vi "Lab Panel V4.86.vi"() -> ()   [LabVIEW 2013] (continued)
                        n565 = Create Folder(path (use dialog)=w897) -> (error out=w896:errorcluster)  [unwired: 2 in, 2 out]
                        n566 = global write "Global 1.vi" "LAB02-1 FILE"(w883) -> ()
                        n567 = call <vilib>:"Clear Errors.vi"("error in (no error)"=w896) -> ()  [unwired: 6 in, 1 out]
                      }
                      frame #1 {
                        (unwired) FALSE
                        n568 = String To Path(string=w907) -> (path=w903:path)
                        n569 = TDMS Open(6:FALSE, 10:T18."create or replace" ("operation (0:open)"), 11:w903) -> (0:w902:errorcluster, 3:→"TDMS LAB02-1":refnum<k34>)  [unwired: 4 in]
                      }
                      frame #2 {
                        n570 = local read "SET LAB02-1"() -> (w913:T5)
                        n571 = local read "TDMS LAB02-1"() -> (w924:refnum<k34>)
                        n572 = Build Array("Testers Name", "Description", "Set Test Cycles", "T-Rise minutes", "T-Rise Deg C") -> (w914:string[])
                        n573 = Unbundle(w913) -> ("NAME"=w912:string, "DESCRIPTION"=w911:string, "CYCLES"=w910:dbl, "T-RISE mins"=w909:dbl, "T-RISE deg C"=w908:dbl)
                        n574 = Number To Decimal String(number=w910) -> (decimal integer string=w923:string)  [unwired: 1 in]
                        n575 = Number To Decimal String(number=w909) -> (decimal integer string=w922:string)  [unwired: 1 in]
                        n576 = Number To Decimal String(number=w908) -> (decimal integer string=w921:string)  [unwired: 1 in]
                        n577 = Build Array(w912, w911, w923, w922, w921) -> (w920:string[])
                        n578 = TDMS Set Properties(5:w920, 7:w914, 11:w924) -> ()  [unwired: 3 in, 4 out]
                      }
                      frame #3 {
                        n579 = local read "DISP LAB02-1"() -> (w929:T4)
                        n580 = Concatenate Strings("LAB02-1  ", w928) -> (w930:string)
                        n581 = Two Button Dialog(message=w930, 1:w926, 2:w927) -> (T button?=w932:bool)
                        n582 = case shown="True" w932 {
                          tunnel: w929 -> [w939 w940]
                          tunnel: [w939 w940] -> w936
                          tunnel: [w938 w941] -> w935
                          tunnel: [w937 w941] -> w934
                          frame False {
                            n583 = Unbundle(w939) -> ("CYCLE"=w938:dbl, "MINS"=w937:dbl)  [unwired: 1 out]
                          }
                          frame True {
                            w941 = 0.0
                          }
                        }
                        n584 = Bundle(cluster=w936, "CYCLE"=w935, "MINS"=w934, "STATUS"="RUN") -> (w925:T4)
                        n585 = local write "DISP LAB02-1"(w925) -> ()
                      }
                      frame #4 {
                        n586 = local read "SIG LAB02-1"() -> (w944:T2)
                        n587 = local read "TEMP START LAB02-1"() -> (w946:cluster{"TL":dbl, "TN":dbl})
                        n588 = Unbundle(w944) -> ("Tmp Live"=w943:dbl, "Tmp Neut"=w942:dbl)  [unwired: 3 out]
                        n589 = Bundle(cluster=w946, "TL"=w943, "TN"=w942) -> (w945:cluster{"TL":dbl, "TN":dbl})
                        n590 = local write "TEMP START LAB02-1"(w945) -> ()
                      }
                    }
                  }
                }
              }
              event "RUN LAB02-2": Value Change {
                n591 = event-data() -> ("NewVal"=w950:bool)  [unwired: 1 in, 5 out]
                n592 = local write "run lab02-2"(w950) -> ()
                n593 = case shown="True" w950 {
                  tunnel: w956 -> [_ w992]
                  tunnel: w955 -> [_ w991]
                  tunnel: w953 -> [w958 w990]
                  tunnel: w954 -> [_ w989]
                  tunnel: w952 -> [_ w988]
                  tunnel: [w957 w987] -> w951
                  tunnel: w949 -> [_ w986]
                  tunnel: w948 -> [_ w985]
                  tunnel: w947 -> [_ w984]
                  frame False {
                    # "stop test"
                    n594 = stacked-sequence {
                      tunnel: w958 -> [w967 _]
                      tunnel: [w959 _] -> w957
                      frame #0 {
                        n595 = local read "DISP LAB02-2"() -> (w966:T4)
                        n596 = Unbundle(w966) -> ("CYCLE"=w964:dbl, "MINS"=w965:dbl)  [unwired: 1 out]
                        n597 = case shown="\"CYCLE TEST\"" w967 {
                          tunnel: w965 -> [_ _ w974]
                          tunnel: w964 -> [w972 w973 _]
                          tunnel: [w972 w973 w974] -> w963
                          frame "CHART TEST", Default {
                          }
                          frame "CYCLE TEST" {
                          }
                          frame "T-RISE TEST" {
                          }
                        }
                        n598 = local read "TDMS LAB02-2"() -> (w971:refnum<k34>)
                        n599 = Build Array("STOPPED") -> (w968:string[])
                        n600 = Build Array(w963) -> (w962:dbl[])
                        n601 = TDMS Write(0:w971, 5:"TEST RESULT", 7:w968, 9:w962) -> (4:w960:refnum<k34>, 15:w961:errorcluster)  [unwired: 2 in, 2 out]
                        n602 = TDMS Close(8:w961, 11:w960) -> (0:w959:errorcluster)  [unwired: 1 out]
                      }
                      frame #1 {
                        n603 = local read "DISP LAB02-2"() -> (w978:T4)
                        n604 = stacked-sequence {
                          tunnel: "LAB02-2" -> [w980 w982]
                          frame #0 {
                            n605 = call "sub vi - defrag tdms v1.vi"("panel id"=w980) -> ("error out"=w979:errorcluster)  [unwired: 10 in]
                            n606 = local write "data file error"(w979) -> ()
                          }
                          frame #1 {
                            n607 = call "Save data file to network drive v2.vi"("panel id"=w982) -> ("network file save error"=w981:errorcluster)  [unwired: 9 in, 1 out]
                            n608 = local write "RESULT LAB02-2"(FALSE) -> ()
                            n609 = local write "data file error"(w981) -> ()
                          }
                        }
                        n610 = Bundle(cluster=w978, "STATUS"="STOP") -> (w976:T4)  [unwired: 2 in]
                        n611 = local write "DISP LAB02-2"(w976) -> ()
                      }
                    }
                  }
                  frame True {
                    # "start new test and create test file"
                    n612 = stacked-sequence {
                      seq-local: [w993 _ _ _ _] -> [_ w1017 _ _ _]
                      tunnel: w992 -> [w998 _ _ _ _]
                      tunnel: w991 -> [w995 _ _ _ _]
                      tunnel: w990 -> [w1008 _ _ _ _]
                      tunnel: w989 -> [w1001 _ _ _ _]
                      tunnel: w988 -> [w996 _ _ _ _]
                      tunnel: [_ w1012 _ _ _] -> w987
                      tunnel: w986 -> [_ _ _ w1038 _]
                      tunnel: w985 -> [_ _ _ w1037 _]
                      tunnel: w984 -> [_ _ _ w1036 _]
                      frame #0 {
                        w994 = "\\"
                        n613 = local read "SET LAB02-2"() -> (w1003:T5)
                        n614 = case shown="\"CYCLE TEST\"" w1008 {
                          tunnel: ["L02-2-CHART TEST-" "L02-2-CYCLE TEST-" "L02-2-T-RISE TEST-"] -> w1004
                          frame "CHART TEST", Default {
                          }
                          frame "CYCLE TEST" {
                          }
                          frame "T-RISE TEST" {
                          }
                        }
                        n615 = Unbundle(w1003) -> ("DESCRIPTION"=w1002:string)  [unwired: 4 out]
                        n616 = Concatenate Strings(w998, "\\", w996, w994, w995, w994) -> (w1005:string)
                        n617 = String To Path(string=w1005) -> (path=w1007:path)
                        n618 = Concatenate Strings(w1005, w1004, w1002, "-", w1001, ".tdms") -> (w993:string)
                        n619 = Create Folder(path (use dialog)=w1007) -> (error out=w1006:errorcluster)  [unwired: 2 in, 2 out]
                        n620 = global write "Global 1.vi" "LAB02-2 FILE"(w993) -> ()
                        n621 = call <vilib>:"Clear Errors.vi"("error in (no error)"=w1006) -> ()  [unwired: 6 in, 1 out]
                      }
                      frame #1 {
                        (unwired) FALSE
                        n622 = String To Path(string=w1017) -> (path=w1013:path)
                        n623 = TDMS Open(6:FALSE, 10:T18."create or replace" ("operation (0:open)"), 11:w1013) -> (0:w1012:errorcluster, 3:→"TDMS LAB02-2":refnum<k34>)  [unwired: 4 in]
                      }
                      frame #2 {
                        n624 = local read "SET LAB02-2"() -> (w1023:T5)
                        n625 = local read "TDMS LAB02-2"() -> (w1034:refnum<k34>)
                        n626 = Build Array("Testers Name", "Description", "Set Test Cycles", "T-Rise minutes", "T-Rise Deg C") -> (w1024:string[])
                        n627 = Unbundle(w1023) -> ("NAME"=w1022:string, "DESCRIPTION"=w1021:string, "CYCLES"=w1020:dbl, "T-RISE mins"=w1019:dbl, "T-RISE deg C"=w1018:dbl)
                        n628 = Number To Decimal String(number=w1020) -> (decimal integer string=w1033:string)  [unwired: 1 in]
                        n629 = Number To Decimal String(number=w1019) -> (decimal integer string=w1032:string)  [unwired: 1 in]
                        n630 = Number To Decimal String(number=w1018) -> (decimal integer string=w1031:string)  [unwired: 1 in]
                        n631 = Build Array(w1022, w1021, w1033, w1032, w1031) -> (w1030:string[])
                        n632 = TDMS Set Properties(5:w1030, 7:w1024, 11:w1034) -> ()  [unwired: 3 in, 4 out]
                      }
                      frame #3 {
                        n633 = local read "DISP LAB02-2"() -> (w1039:T4)
                        n634 = Concatenate Strings("LAB02-2  ", w1038) -> (w1040:string)
                        n635 = Two Button Dialog(message=w1040, 1:w1036, 2:w1037) -> (T button?=w1042:bool)
                        n636 = case shown="True" w1042 {
                          tunnel: w1039 -> [w1049 w1050]
                          tunnel: [w1049 w1050] -> w1046
                          tunnel: [w1048 w1051] -> w1045
                          tunnel: [w1047 w1051] -> w1044
                          frame False {
                            n637 = Unbundle(w1049) -> ("CYCLE"=w1048:dbl, "MINS"=w1047:dbl)  [unwired: 1 out]
                          }
                          frame True {
                            w1051 = 0.0
                          }
                        }
                        n638 = Bundle(cluster=w1046, "CYCLE"=w1045, "MINS"=w1044, "STATUS"="RUN") -> (w1035:T4)
                        n639 = local write "DISP LAB02-2"(w1035) -> ()
                      }
                      frame #4 {
                        n640 = local read "SIG LAB02-2"() -> (w1054:T2)
                        n641 = local read "TEMP START LAB02-2"() -> (w1056:cluster{"TL":dbl, "TN":dbl})
                        n642 = Unbundle(w1054) -> ("Tmp Live"=w1053:dbl, "Tmp Neut"=w1052:dbl)  [unwired: 3 out]
                        n643 = Bundle(cluster=w1056, "TL"=w1053, "TN"=w1052) -> (w1055:cluster{"TL":dbl, "TN":dbl})
                        n644 = local write "TEMP START LAB02-2"(w1055) -> ()
                      }
                    }
                  }
                }
              }
              event "RUN LAB03-1": Value Change {
                n645 = event-data() -> ("NewVal"=w1060:bool)  [unwired: 1 in, 5 out]
                n646 = local write "run lab03-1"(w1060) -> ()
                n647 = case shown="True" w1060 {
                  tunnel: w1066 -> [_ w1102]
                  tunnel: w1065 -> [_ w1101]
                  tunnel: w1063 -> [w1068 w1100]
                  tunnel: w1064 -> [_ w1099]
                  tunnel: w1062 -> [_ w1098]
                  tunnel: [w1067 w1097] -> w1061
                  tunnel: w1059 -> [_ w1096]
                  tunnel: w1058 -> [_ w1095]
                  tunnel: w1057 -> [_ w1094]
                  frame False {
                    # "stop test"
                    n648 = stacked-sequence {
                      tunnel: w1068 -> [w1077 _]
                      tunnel: [w1069 _] -> w1067
                      frame #0 {
                        n649 = local read "DISP LAB03-1"() -> (w1076:T4)
                        n650 = Unbundle(w1076) -> ("CYCLE"=w1074:dbl, "MINS"=w1075:dbl)  [unwired: 1 out]
                        n651 = case shown="\"CYCLE TEST\"" w1077 {
                          tunnel: w1075 -> [_ _ w1084]
                          tunnel: w1074 -> [w1082 w1083 _]
                          tunnel: [w1082 w1083 w1084] -> w1073
                          frame "CHART TEST", Default {
                          }
                          frame "CYCLE TEST" {
                          }
                          frame "T-RISE TEST" {
                          }
                        }
                        n652 = local read "TDMS LAB03-1"() -> (w1081:refnum<k34>)
                        n653 = Build Array("STOPPED") -> (w1078:string[])
                        n654 = Build Array(w1073) -> (w1072:dbl[])
                        n655 = TDMS Write(0:w1081, 5:"TEST RESULT", 7:w1078, 9:w1072) -> (4:w1070:refnum<k34>, 15:w1071:errorcluster)  [unwired: 2 in, 2 out]
                        n656 = TDMS Close(8:w1071, 11:w1070) -> (0:w1069:errorcluster)  [unwired: 1 out]
                      }
                      frame #1 {
                        n657 = local read "DISP LAB03-1"() -> (w1088:T4)
                        n658 = stacked-sequence {
                          tunnel: "LAB03-1" -> [w1090 w1092]
                          frame #0 {
                            n659 = call "sub vi - defrag tdms v1.vi"("panel id"=w1090) -> ("error out"=w1089:errorcluster)  [unwired: 10 in]
                            n660 = local write "data file error"(w1089) -> ()
                          }
                          frame #1 {
                            n661 = call "Save data file to network drive v2.vi"("panel id"=w1092) -> ("network file save error"=w1091:errorcluster)  [unwired: 9 in, 1 out]
                            n662 = local write "RESULT LAB03-1"(FALSE) -> ()
                            n663 = local write "data file error"(w1091) -> ()
                          }
                        }
                        n664 = Bundle(cluster=w1088, "STATUS"="STOP") -> (w1086:T4)  [unwired: 2 in]
                        n665 = local write "DISP LAB03-1"(w1086) -> ()
                      }
                    }
                  }
                  frame True {
                    # "start new test and create test file"
                    n666 = stacked-sequence {
                      seq-local: [w1103 _ _ _ _] -> [_ w1127 _ _ _]
                      tunnel: w1102 -> [w1108 _ _ _ _]
                      tunnel: w1101 -> [w1105 _ _ _ _]
                      tunnel: w1100 -> [w1118 _ _ _ _]
                      tunnel: w1099 -> [w1111 _ _ _ _]
                      tunnel: w1098 -> [w1106 _ _ _ _]
                      tunnel: [_ w1122 _ _ _] -> w1097
                      tunnel: w1096 -> [_ _ _ w1147 _]
                      tunnel: w1095 -> [_ _ _ w1146 _]
                      tunnel: w1094 -> [_ _ _ w1145 _]
                      frame #0 {
                        w1104 = "\\"
                        n667 = local read "SET LAB03-1"() -> (w1113:T5)
                        n668 = case shown="\"T-RISE TEST\"" w1118 {
                          tunnel: ["L03-1-CHART TEST-" "L03-1-CYCLE TEST-" "L03-1-T-RISE TEST-"] -> w1114
                          frame "CHART TEST", Default {
                          }
                          frame "CYCLE TEST" {
                          }
                          frame "T-RISE TEST" {
                          }
                        }
                        n669 = Unbundle(w1113) -> ("DESCRIPTION"=w1112:string)  [unwired: 4 out]
                        n670 = Concatenate Strings(w1108, "\\", w1106, w1104, w1105, w1104) -> (w1115:string)
                        n671 = String To Path(string=w1115) -> (path=w1117:path)
                        n672 = Concatenate Strings(w1115, w1114, w1112, "-", w1111, ".tdms") -> (w1103:string)
                        n673 = Create Folder(path (use dialog)=w1117) -> (error out=w1116:errorcluster)  [unwired: 2 in, 2 out]
                        n674 = global write "Global 1.vi" "LAB03-1 FILE"(w1103) -> ()
                        n675 = call <vilib>:"Clear Errors.vi"("error in (no error)"=w1116) -> ()  [unwired: 6 in, 1 out]
                      }
                      frame #1 {
                        (unwired) FALSE
                        n676 = String To Path(string=w1127) -> (path=w1123:path)
                        n677 = TDMS Open(6:FALSE, 10:T18."create or replace" ("operation (0:open)"), 11:w1123) -> (0:w1122:errorcluster, 3:→"TDMS LAB03-1":refnum<k34>)  [unwired: 4 in]
                      }
                      frame #2 {
                        n678 = local read "SET LAB03-1"() -> (w1133:T5)
                        n679 = local read "TDMS LAB03-1"() -> (w1144:refnum<k34>)
                        n680 = Build Array("Testers Name", "Description", "Set Test Cycles", "T-Rise minutes", "T-Rise Deg C") -> (w1134:string[])
                        n681 = Unbundle(w1133) -> ("NAME"=w1132:string, "DESCRIPTION"=w1131:string, "CYCLES"=w1130:dbl, "T-RISE mins"=w1129:dbl, "T-RISE deg C"=w1128:dbl)
                        n682 = Number To Decimal String(number=w1130) -> (decimal integer string=w1143:string)  [unwired: 1 in]
                        n683 = Number To Decimal String(number=w1129) -> (decimal integer string=w1142:string)  [unwired: 1 in]
                        n684 = Number To Decimal String(number=w1128) -> (decimal integer string=w1141:string)  [unwired: 1 in]
                        n685 = Build Array(w1132, w1131, w1143, w1142, w1141) -> (w1140:string[])
                        n686 = TDMS Set Properties(5:w1140, 7:w1134, 11:w1144) -> ()  [unwired: 3 in, 4 out]
                      }
                      frame #3 {
                        n687 = local read "DISP LAB03-1"() -> (w1149:T4)
                        n688 = Concatenate Strings("LAB03-1  ", w1147) -> (w1150:string)
                        n689 = Two Button Dialog(message=w1150, 1:w1145, 2:w1146) -> (T button?=w1152:bool)
                        n690 = case shown="True" w1152 {
                          tunnel: w1149 -> [w1159 w1160]
                          tunnel: [w1159 w1160] -> w1156
                          tunnel: [w1158 w1161] -> w1155
                          tunnel: [w1157 w1161] -> w1154
                          frame False {
                            n691 = Unbundle(w1159) -> ("CYCLE"=w1158:dbl, "MINS"=w1157:dbl)  [unwired: 1 out]
                          }
                          frame True {
                            w1161 = 0.0
                          }
                        }
                        n692 = Bundle(cluster=w1156, "CYCLE"=w1155, "MINS"=w1154, "STATUS"="RUN") -> (w1148:T4)
                        n693 = local write "DISP LAB03-1"(w1148) -> ()
                      }
                      frame #4 {
                        n694 = local read "SIG LAB03-1"() -> (w1164:T2)
                        n695 = local read "TEMP START LAB03-1"() -> (w1166:cluster{"TL":dbl, "TN":dbl})
                        n696 = Unbundle(w1164) -> ("Tmp Live"=w1163:dbl, "Tmp Neut"=w1162:dbl)  [unwired: 3 out]
                        n697 = Bundle(cluster=w1166, "TL"=w1163, "TN"=w1162) -> (w1165:cluster{"TL":dbl, "TN":dbl})
                        n698 = local write "TEMP START LAB03-1"(w1165) -> ()
                      }
                    }
                  }
                }
              }
              event "RUN LAB03-2": Value Change {
                n699 = event-data() -> ("NewVal"=w1170:bool)  [unwired: 1 in, 5 out]
                n700 = local write "run lab03-2"(w1170) -> ()
                n701 = case shown="True" w1170 {
                  tunnel: w1176 -> [_ w1212]
                  tunnel: w1175 -> [_ w1211]
                  tunnel: w1173 -> [w1178 w1210]
                  tunnel: w1174 -> [_ w1209]
                  tunnel: w1172 -> [_ w1208]
                  tunnel: [w1177 w1207] -> w1171
                  tunnel: w1169 -> [_ w1206]
                  tunnel: w1168 -> [_ w1205]
                  tunnel: w1167 -> [_ w1204]
                  frame False {
                    # "stop test"
                    n702 = stacked-sequence {
                      tunnel: w1178 -> [w1187 _]
                      tunnel: [w1179 _] -> w1177
                      frame #0 {
                        n703 = local read "DISP LAB03-2"() -> (w1186:T4)
                        n704 = Unbundle(w1186) -> ("CYCLE"=w1184:dbl, "MINS"=w1185:dbl)  [unwired: 1 out]
                        n705 = case shown="\"CYCLE TEST\"" w1187 {
                          tunnel: w1185 -> [_ _ w1194]
                          tunnel: w1184 -> [w1192 w1193 _]
                          tunnel: [w1192 w1193 w1194] -> w1183
                          frame "CHART TEST", Default {
                          }
                          frame "CYCLE TEST" {
                          }
                          frame "T-RISE TEST" {
                          }
                        }
                        n706 = local read "TDMS LAB03-2"() -> (w1191:refnum<k34>)
                        n707 = Build Array("STOPPED") -> (w1188:string[])
                        n708 = Build Array(w1183) -> (w1182:dbl[])
                        n709 = TDMS Write(0:w1191, 5:"TEST RESULT", 7:w1188, 9:w1182) -> (4:w1180:refnum<k34>, 15:w1181:errorcluster)  [unwired: 2 in, 2 out]
                        n710 = TDMS Close(8:w1181, 11:w1180) -> (0:w1179:errorcluster)  [unwired: 1 out]
                      }
                      frame #1 {
                        n711 = local read "DISP LAB03-2"() -> (w1198:T4)
                        n712 = stacked-sequence {
                          tunnel: "LAB03-2" -> [w1200 w1202]
                          frame #0 {
                            n713 = call "sub vi - defrag tdms v1.vi"("panel id"=w1200) -> ("error out"=w1199:errorcluster)  [unwired: 10 in]
                            n714 = local write "data file error"(w1199) -> ()
                          }
                          frame #1 {
                            n715 = call "Save data file to network drive v2.vi"("panel id"=w1202) -> ("network file save error"=w1201:errorcluster)  [unwired: 9 in, 1 out]
                            n716 = local write "RESULT LAB03-2"(FALSE) -> ()
                            n717 = local write "data file error"(w1201) -> ()
                          }
                        }
                        n718 = Bundle(cluster=w1198, "STATUS"="STOP") -> (w1196:T4)  [unwired: 2 in]
                        n719 = local write "DISP LAB03-2"(w1196) -> ()
                      }
                    }
                  }
                  frame True {
                    # "start new test and create test file"
                    n720 = stacked-sequence {
                      seq-local: [w1213 _ _ _ _] -> [_ w1237 _ _ _]
                      tunnel: w1212 -> [w1218 _ _ _ _]
                      tunnel: w1211 -> [w1215 _ _ _ _]
                      tunnel: w1210 -> [w1228 _ _ _ _]
                      tunnel: w1209 -> [w1221 _ _ _ _]
                      tunnel: w1208 -> [w1216 _ _ _ _]
                      tunnel: [_ w1232 _ _ _] -> w1207
                      tunnel: w1206 -> [_ _ _ w1258 _]
                      tunnel: w1205 -> [_ _ _ w1257 _]
                      tunnel: w1204 -> [_ _ _ w1256 _]
                      frame #0 {
                        w1214 = "\\"
                        n721 = local read "SET LAB03-2"() -> (w1223:T5)
                        n722 = case shown="\"T-RISE TEST\"" w1228 {
                          tunnel: ["L03-2-CHART TEST-" "L03-2-CYCLE TEST-" "L03-2-T-RISE TEST-"] -> w1224
                          frame "CHART TEST", Default {
                          }
                          frame "CYCLE TEST" {
                          }
                          frame "T-RISE TEST" {
                          }
                        }
                        n723 = Unbundle(w1223) -> ("DESCRIPTION"=w1222:string)  [unwired: 4 out]
                        n724 = Concatenate Strings(w1218, "\\", w1216, w1214, w1215, w1214) -> (w1225:string)
                        n725 = String To Path(string=w1225) -> (path=w1227:path)
                        n726 = Concatenate Strings(w1225, w1224, w1222, "-", w1221, ".tdms") -> (w1213:string)
                        n727 = Create Folder(path (use dialog)=w1227) -> (error out=w1226:errorcluster)  [unwired: 2 in, 2 out]
                        n728 = global write "Global 1.vi" "LAB03-2 FILE"(w1213) -> ()
                        n729 = call <vilib>:"Clear Errors.vi"("error in (no error)"=w1226) -> ()  [unwired: 6 in, 1 out]
                      }
                      frame #1 {
                        (unwired) FALSE
                        n730 = String To Path(string=w1237) -> (path=w1233:path)
                        n731 = TDMS Open(6:FALSE, 10:T18."create or replace" ("operation (0:open)"), 11:w1233) -> (0:w1232:errorcluster, 3:→"TDMS LAB03-2":refnum<k34>)  [unwired: 4 in]
                      }
                      frame #2 {
                        n732 = local read "SET LAB03-2"() -> (w1243:T5)
                        n733 = local read "TDMS LAB03-2"() -> (w1254:refnum<k34>)
                        n734 = Build Array("Testers Name", "Description", "Set Test Cycles", "T-Rise minutes", "T-Rise Deg C") -> (w1244:string[])
                        n735 = Unbundle(w1243) -> ("NAME"=w1242:string, "DESCRIPTION"=w1241:string, "CYCLES"=w1240:dbl, "T-RISE mins"=w1239:dbl, "T-RISE deg C"=w1238:dbl)
                        n736 = Number To Decimal String(number=w1240) -> (decimal integer string=w1253:string)  [unwired: 1 in]
                        n737 = Number To Decimal String(number=w1239) -> (decimal integer string=w1252:string)  [unwired: 1 in]
                        n738 = Number To Decimal String(number=w1238) -> (decimal integer string=w1251:string)  [unwired: 1 in]
                        n739 = Build Array(w1242, w1241, w1253, w1252, w1251) -> (w1250:string[])
                        n740 = TDMS Set Properties(5:w1250, 7:w1244, 11:w1254) -> ()  [unwired: 3 in, 4 out]
                      }
                      frame #3 {
                        n741 = local read "DISP LAB03-2"() -> (w1259:T4)
                        n742 = Concatenate Strings("LAB03-2  ", w1258) -> (w1260:string)
                        n743 = Two Button Dialog(message=w1260, 1:w1256, 2:w1257) -> (T button?=w1262:bool)
                        n744 = case shown="True" w1262 {
                          tunnel: w1259 -> [w1269 w1270]
                          tunnel: [w1269 w1270] -> w1266
                          tunnel: [w1268 w1271] -> w1265
                          tunnel: [w1267 w1271] -> w1264
                          frame False {
                            n745 = Unbundle(w1269) -> ("CYCLE"=w1268:dbl, "MINS"=w1267:dbl)  [unwired: 1 out]
                          }
                          frame True {
                            w1271 = 0.0
                          }
                        }
                        n746 = Bundle(cluster=w1266, "CYCLE"=w1265, "MINS"=w1264, "STATUS"="RUN") -> (w1255:T4)
                        n747 = local write "DISP LAB03-2"(w1255) -> ()
                      }
                      frame #4 {
                        n748 = local read "SIG LAB03-2"() -> (w1274:T2)
                        n749 = local read "TEMP START LAB03-2"() -> (w1276:cluster{"TL":dbl, "TN":dbl})
                        n750 = Unbundle(w1274) -> ("Tmp Live"=w1273:dbl, "Tmp Neut"=w1272:dbl)  [unwired: 3 out]
                        n751 = Bundle(cluster=w1276, "TL"=w1273, "TN"=w1272) -> (w1275:cluster{"TL":dbl, "TN":dbl})
                        n752 = local write "TEMP START LAB03-2"(w1275) -> ()
                      }
                    }
                  }
                }
              }
              event "RUN LAB04-1": Value Change {
                n753 = event-data() -> ("NewVal"=w1280:bool)  [unwired: 1 in, 5 out]
                n754 = local write "run lab04-1"(w1280) -> ()
                n755 = case shown="True" w1280 {
                  tunnel: w1286 -> [_ w1322]
                  tunnel: w1285 -> [_ w1321]
                  tunnel: w1283 -> [w1288 w1320]
                  tunnel: w1284 -> [_ w1319]
                  tunnel: w1282 -> [_ w1318]
                  tunnel: [w1287 w1317] -> w1281
                  tunnel: w1279 -> [_ w1316]
                  tunnel: w1278 -> [_ w1315]
                  tunnel: w1277 -> [_ w1314]
                  frame False {
                    # "stop test"
                    n756 = stacked-sequence {
                      tunnel: w1288 -> [w1297 _]
                      tunnel: [w1289 _] -> w1287
                      frame #0 {
                        n757 = local read "DISP LAB04-1"() -> (w1296:T4)
                        n758 = Unbundle(w1296) -> ("CYCLE"=w1294:dbl, "MINS"=w1295:dbl)  [unwired: 1 out]
                        n759 = case shown="\"CYCLE TEST\"" w1297 {
                          tunnel: w1295 -> [_ _ w1304]
                          tunnel: w1294 -> [w1302 w1303 _]
                          tunnel: [w1302 w1303 w1304] -> w1293
                          frame "CHART TEST", Default {
                          }
                          frame "CYCLE TEST" {
                          }
                          frame "T-RISE TEST" {
                          }
                        }
                        n760 = local read "TDMS LAB04-1"() -> (w1301:refnum<k34>)
                        n761 = Build Array("STOPPED") -> (w1298:string[])
                        n762 = Build Array(w1293) -> (w1292:dbl[])
                        n763 = TDMS Write(0:w1301, 5:"TEST RESULT", 7:w1298, 9:w1292) -> (4:w1290:refnum<k34>, 15:w1291:errorcluster)  [unwired: 2 in, 2 out]
                        n764 = TDMS Close(8:w1291, 11:w1290) -> (0:w1289:errorcluster)  [unwired: 1 out]
                      }
                      frame #1 {
                        n765 = local read "DISP LAB04-1"() -> (w1308:T4)
                        n766 = stacked-sequence {
                          tunnel: "LAB04-1" -> [w1310 w1312]
                          frame #0 {
                            n767 = call "sub vi - defrag tdms v1.vi"("panel id"=w1310) -> ("error out"=w1309:errorcluster)  [unwired: 10 in]
                            n768 = local write "data file error"(w1309) -> ()
                          }
                          frame #1 {
                            n769 = call "Save data file to network drive v2.vi"("panel id"=w1312) -> ("network file save error"=w1311:errorcluster)  [unwired: 9 in, 1 out]
                            n770 = local write "RESULT LAB04-1"(FALSE) -> ()
                            n771 = local write "data file error"(w1311) -> ()
                          }
                        }
                        n772 = Bundle(cluster=w1308, "STATUS"="STOP") -> (w1306:T4)  [unwired: 2 in]
                        n773 = local write "DISP LAB04-1"(w1306) -> ()
                      }
                    }
                  }
                  frame True {
                    # "start new test and create test file"
                    n774 = stacked-sequence {
                      seq-local: [w1323 _ _ _ _] -> [_ w1347 _ _ _]
                      tunnel: w1322 -> [w1328 _ _ _ _]
                      tunnel: w1321 -> [w1324 _ _ _ _]
                      tunnel: w1320 -> [w1338 _ _ _ _]
                      tunnel: w1319 -> [w1331 _ _ _ _]
                      tunnel: w1318 -> [w1326 _ _ _ _]
                      tunnel: [_ w1342 _ _ _] -> w1317
                      tunnel: w1316 -> [_ _ _ w1368 _]
                      tunnel: w1315 -> [_ _ _ w1367 _]
                      tunnel: w1314 -> [_ _ _ w1366 _]
                      frame #0 {
                        w1325 = "\\"
                        n775 = local read "SET LAB04-1"() -> (w1333:T5)
                        n776 = case shown="\"CYCLE TEST\"" w1338 {
                          tunnel: ["L04-1-CHART TEST-" "L04-1-CYCLE TEST-" "L04-1-T-RISE TEST-"] -> w1334
                          frame "CHART TEST", Default {
                          }
                          frame "CYCLE TEST" {
                          }
                          frame "T-RISE TEST" {
                          }
                        }
                        n777 = Unbundle(w1333) -> ("DESCRIPTION"=w1332:string)  [unwired: 4 out]
                        n778 = Concatenate Strings(w1328, "\\", w1326, w1325, w1324, w1325) -> (w1335:string)
                        n779 = String To Path(string=w1335) -> (path=w1337:path)
                        n780 = Concatenate Strings(w1335, w1334, w1332, "-", w1331, ".tdms") -> (w1323:string)
                        n781 = Create Folder(path (use dialog)=w1337) -> (error out=w1336:errorcluster)  [unwired: 2 in, 2 out]
                        n782 = global write "Global 1.vi" "LAB04-1 FILE"(w1323) -> ()
                        n783 = call <vilib>:"Clear Errors.vi"("error in (no error)"=w1336) -> ()  [unwired: 6 in, 1 out]
                      }
                      frame #1 {
                        (unwired) FALSE
                        n784 = String To Path(string=w1347) -> (path=w1343:path)
                        n785 = TDMS Open(6:FALSE, 10:T18."create or replace" ("operation (0:open)"), 11:w1343) -> (0:w1342:errorcluster, 3:→"TDMS LAB04-1":refnum<k34>)  [unwired: 4 in]
                      }
                      frame #2 {
                        n786 = local read "SET LAB04-1"() -> (w1353:T5)
                        n787 = local read "TDMS LAB04-1"() -> (w1364:refnum<k34>)
                        n788 = Build Array("Testers Name", "Description", "Set Test Cycles", "T-Rise minutes", "T-Rise Deg C") -> (w1354:string[])
                        n789 = Unbundle(w1353) -> ("NAME"=w1352:string, "DESCRIPTION"=w1351:string, "CYCLES"=w1350:dbl, "T-RISE mins"=w1349:dbl, "T-RISE deg C"=w1348:dbl)
                        n790 = Number To Decimal String(number=w1350) -> (decimal integer string=w1363:string)  [unwired: 1 in]
                        n791 = Number To Decimal String(number=w1349) -> (decimal integer string=w1362:string)  [unwired: 1 in]
                        n792 = Number To Decimal String(number=w1348) -> (decimal integer string=w1361:string)  [unwired: 1 in]
                        n793 = Build Array(w1352, w1351, w1363, w1362, w1361) -> (w1360:string[])
                        n794 = TDMS Set Properties(5:w1360, 7:w1354, 11:w1364) -> ()  [unwired: 3 in, 4 out]
                      }
                      frame #3 {
                        n795 = local read "DISP LAB04-1"() -> (w1369:T4)
                        n796 = Concatenate Strings("LAB04-1  ", w1368) -> (w1370:string)
                        n797 = Two Button Dialog(message=w1370, 1:w1366, 2:w1367) -> (T button?=w1372:bool)
                        n798 = case shown="True" w1372 {
                          tunnel: w1369 -> [w1379 w1380]
                          tunnel: [w1379 w1380] -> w1376
                          tunnel: [w1378 w1381] -> w1375
                          tunnel: [w1377 w1381] -> w1374
                          frame False {
                            n799 = Unbundle(w1379) -> ("CYCLE"=w1378:dbl, "MINS"=w1377:dbl)  [unwired: 1 out]
                          }
                          frame True {
                            w1381 = 0.0
                          }
                        }
                        n800 = Bundle(cluster=w1376, "CYCLE"=w1375, "MINS"=w1374, "STATUS"="RUN") -> (w1365:T4)
                        n801 = local write "DISP LAB04-1"(w1365) -> ()
                      }
                      frame #4 {
                        n802 = local read "SIG LAB04-1"() -> (w1384:T2)
                        n803 = local read "TEMP START LAB04-1"() -> (w1386:cluster{"TL":dbl, "TN":dbl})
                        n804 = Unbundle(w1384) -> ("Tmp Live"=w1383:dbl, "Tmp Neut"=w1382:dbl)  [unwired: 3 out]
                        n805 = Bundle(cluster=w1386, "TL"=w1383, "TN"=w1382) -> (w1385:cluster{"TL":dbl, "TN":dbl})
                        n806 = local write "TEMP START LAB04-1"(w1385) -> ()
                      }
                    }
                  }
                }
              }
              event "RUN LAB04-2": Value Change {
                n807 = event-data() -> ("NewVal"=w1390:bool)  [unwired: 1 in, 5 out]
                n808 = local write "run lab04-2"(w1390) -> ()
                n809 = case shown="True" w1390 {
                  tunnel: w1396 -> [_ w1432]
                  tunnel: w1395 -> [_ w1431]
                  tunnel: w1393 -> [w1398 w1430]
                  tunnel: w1394 -> [_ w1429]
                  tunnel: w1392 -> [_ w1428]
                  tunnel: [w1397 w1427] -> w1391
                  tunnel: w1389 -> [_ w1426]
                  tunnel: w1388 -> [_ w1425]
                  tunnel: w1387 -> [_ w1424]
                  frame False {
                    # "stop test"
                    n810 = stacked-sequence {
                      tunnel: w1398 -> [w1407 _]
                      tunnel: [w1399 _] -> w1397
                      frame #0 {
                        n811 = local read "DISP LAB04-2"() -> (w1406:T4)
                        n812 = Unbundle(w1406) -> ("CYCLE"=w1404:dbl, "MINS"=w1405:dbl)  [unwired: 1 out]
                        n813 = case shown="\"CYCLE TEST\"" w1407 {
                          tunnel: w1405 -> [_ _ w1414]
                          tunnel: w1404 -> [w1412 w1413 _]
                          tunnel: [w1412 w1413 w1414] -> w1403
                          frame "CHART TEST", Default {
                          }
                          frame "CYCLE TEST" {
                          }
                          frame "T-RISE TEST" {
                          }
                        }
                        n814 = local read "TDMS LAB04-2"() -> (w1411:refnum<k34>)
                        n815 = Build Array("STOPPED") -> (w1408:string[])
                        n816 = Build Array(w1403) -> (w1402:dbl[])
                        n817 = TDMS Write(0:w1411, 5:"TEST RESULT", 7:w1408, 9:w1402) -> (4:w1400:refnum<k34>, 15:w1401:errorcluster)  [unwired: 2 in, 2 out]
                        n818 = TDMS Close(8:w1401, 11:w1400) -> (0:w1399:errorcluster)  [unwired: 1 out]
                      }
                      frame #1 {
                        n819 = local read "DISP LAB04-2"() -> (w1418:T4)
                        n820 = stacked-sequence {
                          tunnel: "LAB04-2" -> [w1420 w1422]
                          frame #0 {
                            n821 = call "sub vi - defrag tdms v1.vi"("panel id"=w1420) -> ("error out"=w1419:errorcluster)  [unwired: 10 in]
                            n822 = local write "data file error"(w1419) -> ()
                          }
                          frame #1 {
                            n823 = call "Save data file to network drive v2.vi"("panel id"=w1422) -> ("network file save error"=w1421:errorcluster)  [unwired: 9 in, 1 out]
                            n824 = local write "RESULT LAB04-2"(FALSE) -> ()
                            n825 = local write "data file error"(w1421) -> ()
                          }
                        }
                        n826 = Bundle(cluster=w1418, "STATUS"="STOP") -> (w1416:T4)  [unwired: 2 in]
                        n827 = local write "DISP LAB04-2"(w1416) -> ()
                      }
                    }
                  }
                  frame True {
                    # "start new test and create test file"
                    n828 = stacked-sequence {
                      seq-local: [w1433 _ _ _ _] -> [_ w1457 _ _ _]
                      tunnel: w1432 -> [w1438 _ _ _ _]
                      tunnel: w1431 -> [w1434 _ _ _ _]
                      tunnel: w1430 -> [w1448 _ _ _ _]
                      tunnel: w1429 -> [w1441 _ _ _ _]
                      tunnel: w1428 -> [w1436 _ _ _ _]
                      tunnel: [_ w1452 _ _ _] -> w1427
                      tunnel: w1426 -> [_ _ _ w1478 _]
                      tunnel: w1425 -> [_ _ _ w1477 _]
                      tunnel: w1424 -> [_ _ _ w1476 _]
                      frame #0 {
                        w1435 = "\\"
                        n829 = local read "SET LAB04-2"() -> (w1443:T5)
                        n830 = case shown="\"CHART TEST\", Default" w1448 {
                          tunnel: ["L04-2-CHART TEST-" "L04-2-CYCLE TEST-" "L04-2-T-RISE TEST-"] -> w1444
                          frame "CHART TEST", Default {
                          }
                          frame "CYCLE TEST" {
                          }
                          frame "T-RISE TEST" {
                          }
                        }
                        n831 = Unbundle(w1443) -> ("DESCRIPTION"=w1442:string)  [unwired: 4 out]
                        n832 = Concatenate Strings(w1438, "\\", w1436, w1435, w1434, w1435) -> (w1445:string)
                        n833 = String To Path(string=w1445) -> (path=w1447:path)
                        n834 = Concatenate Strings(w1445, w1444, w1442, "-", w1441, ".tdms") -> (w1433:string)
                        n835 = Create Folder(path (use dialog)=w1447) -> (error out=w1446:errorcluster)  [unwired: 2 in, 2 out]
                        n836 = global write "Global 1.vi" "LAB04-2 FILE"(w1433) -> ()
                        n837 = call <vilib>:"Clear Errors.vi"("error in (no error)"=w1446) -> ()  [unwired: 6 in, 1 out]
                      }
                      frame #1 {
                        (unwired) FALSE
                        n838 = String To Path(string=w1457) -> (path=w1453:path)
                        n839 = TDMS Open(6:FALSE, 10:T18."create or replace" ("operation (0:open)"), 11:w1453) -> (0:w1452:errorcluster, 3:→"TDMS LAB04-2":refnum<k34>)  [unwired: 4 in]
                      }
                      frame #2 {
                        n840 = local read "SET LAB04-2"() -> (w1463:T5)
                        n841 = local read "TDMS LAB04-2"() -> (w1474:refnum<k34>)
                        n842 = Build Array("Testers Name", "Description", "Set Test Cycles", "T-Rise minutes", "T-Rise Deg C") -> (w1464:string[])
                        n843 = Unbundle(w1463) -> ("NAME"=w1462:string, "DESCRIPTION"=w1461:string, "CYCLES"=w1460:dbl, "T-RISE mins"=w1459:dbl, "T-RISE deg C"=w1458:dbl)
                        n844 = Number To Decimal String(number=w1460) -> (decimal integer string=w1473:string)  [unwired: 1 in]
                        n845 = Number To Decimal String(number=w1459) -> (decimal integer string=w1472:string)  [unwired: 1 in]
                        n846 = Number To Decimal String(number=w1458) -> (decimal integer string=w1471:string)  [unwired: 1 in]
                        n847 = Build Array(w1462, w1461, w1473, w1472, w1471) -> (w1470:string[])
                        n848 = TDMS Set Properties(5:w1470, 7:w1464, 11:w1474) -> ()  [unwired: 3 in, 4 out]
                      }
                      frame #3 {
                        n849 = local read "DISP LAB04-2"() -> (w1479:T4)
                        n850 = Concatenate Strings("LAB04-2 ", w1478) -> (w1480:string)
                        n851 = Two Button Dialog(message=w1480, 1:w1476, 2:w1477) -> (T button?=w1482:bool)
                        n852 = case shown="True" w1482 {
                          tunnel: w1479 -> [w1489 w1490]
                          tunnel: [w1489 w1490] -> w1486
                          tunnel: [w1488 w1491] -> w1485
                          tunnel: [w1487 w1491] -> w1484
                          frame False {
                            n853 = Unbundle(w1489) -> ("CYCLE"=w1488:dbl, "MINS"=w1487:dbl)  [unwired: 1 out]
                          }
                          frame True {
                            w1491 = 0.0
                          }
                        }
                        n854 = Bundle(cluster=w1486, "CYCLE"=w1485, "MINS"=w1484, "STATUS"="RUN") -> (w1475:T4)
                        n855 = local write "DISP LAB04-2"(w1475) -> ()
                      }
                      frame #4 {
                        n856 = local read "SIG LAB04-2"() -> (w1494:T2)
                        n857 = local read "TEMP START LAB04-2"() -> (w1496:cluster{"TL":dbl, "TN":dbl})
                        n858 = Unbundle(w1494) -> ("Tmp Live"=w1493:dbl, "Tmp Neut"=w1492:dbl)  [unwired: 3 out]
                        n859 = Bundle(cluster=w1496, "TL"=w1493, "TN"=w1492) -> (w1495:cluster{"TL":dbl, "TN":dbl})
                        n860 = local write "TEMP START LAB04-2"(w1495) -> ()
                      }
                    }
                  }
                }
              }
              event "RUN LAB05-1": Value Change {
                n861 = event-data() -> ("NewVal"=w1500:bool)  [unwired: 1 in, 5 out]
                n862 = local write "run lab05-1"(w1500) -> ()
                n863 = case shown="True" w1500 {
                  tunnel: w1506 -> [_ w1542]
                  tunnel: w1505 -> [_ w1541]
                  tunnel: w1503 -> [w1508 w1540]
                  tunnel: w1504 -> [_ w1539]
                  tunnel: w1502 -> [_ w1538]
                  tunnel: [w1507 w1537] -> w1501
                  tunnel: w1499 -> [_ w1536]
                  tunnel: w1498 -> [_ w1535]
                  tunnel: w1497 -> [_ w1534]
                  frame False {
                    # "stop test"
                    n864 = stacked-sequence {
                      tunnel: w1508 -> [w1517 _]
                      tunnel: [w1509 _] -> w1507
                      frame #0 {
                        n865 = local read "DISP LAB05-1"() -> (w1516:T4)
                        n866 = Unbundle(w1516) -> ("CYCLE"=w1514:dbl, "MINS"=w1515:dbl)  [unwired: 1 out]
                        n867 = case shown="\"CYCLE TEST\"" w1517 {
                          tunnel: w1515 -> [_ _ w1524]
                          tunnel: w1514 -> [w1522 w1523 _]
                          tunnel: [w1522 w1523 w1524] -> w1513
                          frame "CHART TEST", Default {
                          }
                          frame "CYCLE TEST" {
                          }
                          frame "T-RISE TEST" {
                          }
                        }
                        n868 = local read "TDMS LAB05-1"() -> (w1521:refnum<k34>)
                        n869 = Build Array("STOPPED") -> (w1518:string[])
                        n870 = Build Array(w1513) -> (w1512:dbl[])
                        n871 = TDMS Write(0:w1521, 5:"TEST RESULT", 7:w1518, 9:w1512) -> (4:w1510:refnum<k34>, 15:w1511:errorcluster)  [unwired: 2 in, 2 out]
                        n872 = TDMS Close(8:w1511, 11:w1510) -> (0:w1509:errorcluster)  [unwired: 1 out]
                      }
                      frame #1 {
                        n873 = local read "DISP LAB05-1"() -> (w1528:T4)
                        n874 = stacked-sequence {
                          tunnel: "LAB05-1" -> [w1530 w1532]
                          frame #0 {
                            n875 = call "sub vi - defrag tdms v1.vi"("panel id"=w1530) -> ("error out"=w1529:errorcluster)  [unwired: 10 in]
                            n876 = local write "data file error"(w1529) -> ()
                          }
                          frame #1 {
                            n877 = call "Save data file to network drive v2.vi"("panel id"=w1532) -> ("network file save error"=w1531:errorcluster)  [unwired: 9 in, 1 out]
                            n878 = local write "RESULT LAB05-1"(FALSE) -> ()
                            n879 = local write "data file error"(w1531) -> ()
                          }
                        }
                        n880 = Bundle(cluster=w1528, "STATUS"="STOP") -> (w1526:T4)  [unwired: 2 in]
                        n881 = local write "DISP LAB05-1"(w1526) -> ()
                      }
                    }
                  }
                  frame True {
                    # "start new test and create test file"
